vi "Wrap in Brackets.vi"(11 "String":string) -> (3 "String with Brackets":string)   [LabVIEW 2015, in "NI_JSON Parsing.lvlib"]
uses:
  NI_JSON Parsing.lvlib
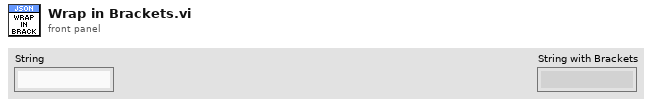
[diagram p1: front panel]
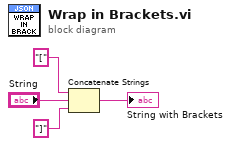
[diagram p0: block diagram]
diagram:
  n1 = Concatenate Strings("[", "String", "]") -> (→"String with Brackets":string)
